vi "RESTful Escape VI Section Name.vi"(9 "error in":errorcluster, 10 "Label.Text":string) -> (1 "error out":errorcluster, 2 "result string":string)   [LabVIEW 2020]
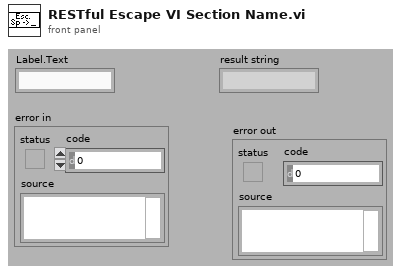
[diagram p1: front panel]
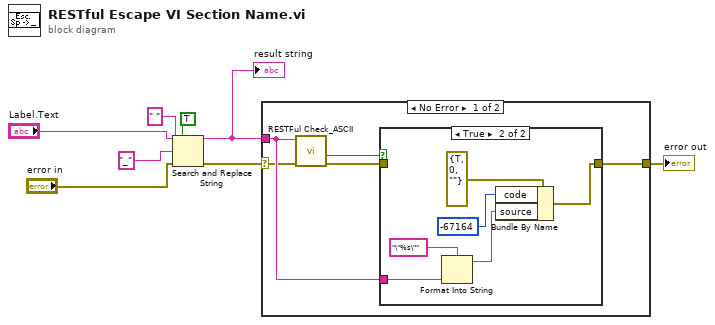
[diagram p0: block diagram]
diagram:
  n1 = Search and Replace String(replace all?=TRUE ("replace all? (F)"), input string="Label.Text", search string=" ", replace string="_" ("replace string (\"\")"), error in="error in") -> (result string=w3:string, error out=w1:errorcluster)  [unwired: 5 out]
  "result string" <- w3
  n2 = case shown="No Error" w1 {
    selector: w1 -> [w9 w21]
    tunnel: w3 -> [w11 _]
    tunnel: [w10 w21] -> w2
    frame No Error {
      n3 = call <vilib>:"RESTFul Check_ASCII.vi"("error in (no error)"=w9, "string in"=w11) -> ("error out"=w12:errorcluster, "invalid chars?"=w13:bool)  [unwired: 8 out]
      n4 = case shown="True" w13 {
        tunnel: w12 -> [w14 _]
        tunnel: [w14 w18] -> w10
        tunnel: w11 -> [_ w15]
        frame False {
        }
        frame True {
          n5 = Format Into String(format string="\"%s\"", w15) -> (resulting string=w16:string)  [unwired: 2 in, 1 out]
          n6 = Bundle By Name(cluster=errorcluster {"status"=TRUE, "code"=0, "source"=""} ("error in (no error)"), "code"=-67164 ("error code (0)"), "source"=w16) -> (w18:errorcluster)
        }
      }
    }
    frame Error {
    }
  }
  "error out" <- w2
